vi "소숫점 2자리.vi"(11 "input Value":dbl) -> (3 "output value":dbl)   [LabVIEW 2019]
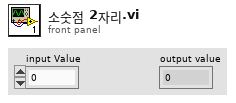
[diagram p1: front panel]
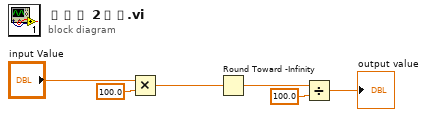
[diagram p0: block diagram]
diagram:
  n1 = Multiply(x="input Value", y=100.0) -> (x*y=w3:dbl)
  n2 = Round Toward -Infinity(1:w3) -> (0:w4:dbl)
  n3 = Divide(x=w4, y=100.0) -> (x/y=→"output value":dbl)
